vi "LSX Set Gripper.vi"(6 "s2":i32, 7 "c2":i32, 8 "error in (no error)":errorcluster, 9 "s1":i32, 10 "c1":i32, 11 "lLSID":i32) -> (0 "error out":errorcluster, 3 "function return":i32)   [LabVIEW 2018, in "Tango.lvlib"]
doc: "TANGOAPI int TANGOCALL LSX_SetGripper (int lLSID, int c1, int s1, int c2, int s2);"
uses:
  Tango.lvlib
  SubVIs/Tango_DLL.dll
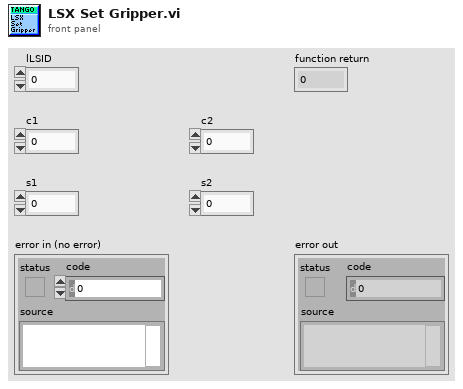
[diagram p1: front panel]
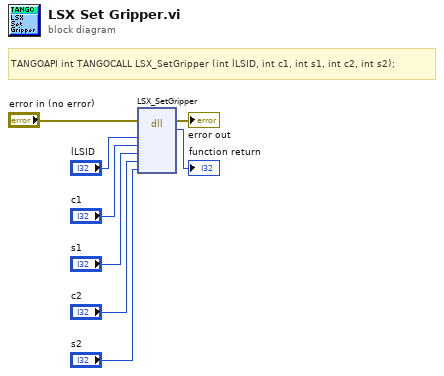
[diagram p0: block diagram]
diagram:
  # "TANGOAPI int TANGOCALL LSX_SetGripper (int lLSID, int c1, int s1, int c2, int s2);"
  n1 = dll-call lib="C:/Users/Familie/Documents/LabviewIX81/lib/TANGO Stage/SubVIs/Tango_DLL.*" fn="LSX_SetGripper"(error in="error in (no error)", "lLSID"="lLSID", "c1"="c1", "s1"="s1", "c2"="c2", "s2"="s2") -> (error out=→"error out":errorcluster, →"function return":i32)  [unwired: 7 in, 1 out]
